vi "Calibration_user_input.vi"(4 "data mode":enum16{"Take new data point", "Refit Curve"}(ring), 6 "Mode":T4, 7 "Fixed n":bool, 8 "OK":T13, 9 "Sampling speeds":T5={"Samples /ch"=300, "Sampling Rate /ch (Hz)"=50.0} {"Sampling Rate /ch (Hz)" min=0 format="%.2f"; "Samples /ch" min=0 step=1}) -> (1 "Sampling speeds Output":T5={"Samples /ch"=300, "Sampling Rate /ch (Hz)"=50.0} {"Sampling Rate /ch (Hz)" min=0 format="%.2f"; "Samples /ch" min=0 step=1}, 2 "Fixed n out":bool, 3 "Temp (deg C)":dbl=21.0 format="%.1f", 5 "Abs Press (mbar)":dbl=1013.0 format="%.1f")   [LabVIEW 2012]
uses:
  Controls/ok_button.ctl
  Controls/Cal_Inst_type.ctl
  Calib_setup.ctl
  Controls/Ref_Inst_type.ctl
  Calib_mode.ctl
  Controls/PWA_Data.ctl
  File/Setup_Filetype.ctl
  Controls/Inst_type.ctl
  ADAM Client/Sub VIs/ADAM Controls/Channel_names.ctl
  Controls/LDA_Setup.ctl
  Controls/Setup.ctl
  Globals/Calib_global.vi
  Globals/Meas_global.vi
  Globals/LDA_meas_global_1.vi
  Globals/LDA_meas_global_2.vi
panel:
  in  "Acquisition Plug in":u16(ring) items=["ADAM_Server_Channels.vi", "DataTranslation.vi", "LDA_IP_DataTranslation.vi", "LDA_IP_NI-DAQmx.vi", "NI-DAQmx.vi", "Simulate_kernal.vi"]
  in  "PWA Data":T1
  in  "Preston tube diammeter in mm":dbl min=0.0
  in  "Reference instrument Orig":T3={"high limit (10V)"=4.0, "low limit (-10V)"=0.0, "Ch No"=4, "Off ch no"=0, "Calib filename"=path "", "Ref Instrument type"=enum."Enter Value"} {"Off ch no" min=0 max=1; "Ch No" min=0 max=7; "low limit (-10V)" min=-10 max=10 format="%.1f"; "high limit (10V)" min=-10 max=10 format="%.1f"}
  out "Message":string
  in  "Ref Instrument type":T2
  out "Info":string
  out "XW Angle Calib Present?":bool
  out "XW Velocity Calib Present?":bool
  in  "Edit temp and Press":bool
  out "2nd ref instrument":T6={"2nd Ref type"=enum."LDA", "2nd inst present"=TRUE}
  in  "Ref vel for angle calib":T7={"high limit (10V)"=6.0, "low limit (-10V)"=0.0, "Ch No"=4, "Off ch no"=0, "Calib filename"=path "", "Ref Instrument type"=enum."LDA"} {"Off ch no" min=0 max=1; "Ch No" min=0 max=50; "low limit (-10V)" min=-10 max=10 format="%.1f"; "high limit (10V)" min=-10 max=10 format="%.1f"}
  out "Instrument type":T8=enum."Cross wire angle"
  in  "angle calib":T9(ring)
  in  "Reference instrument":T7={"high limit (10V)"=4.0, "low limit (-10V)"=0.0, "Ch No"=4, "Off ch no"=0, "Calib filename"=path "", "Ref Instrument type"=enum."Enter Value"} {"Off ch no" min=0 max=1; "Ch No" min=0 max=50; "low limit (-10V)" min=-10 max=10 format="%.1f"; "high limit (10V)" min=-10 max=10 format="%.1f"}
  in  "instrument to calibrate":T10(array[cluster])=[{"high limit (10V)"=5.0, "low limit (-10V)"=3.0, "Ch No"=1, "Off ch no"=1}, {"high limit (10V)"=5.0, "low limit (-10V)"=3.0, "Ch No"=2, "Off ch no"=1}] {"Off ch no" min=0 max=1; "Ch No" min=0 max=1000; "low limit (-10V)" min=-10 max=10 format="%.3f"; "high limit (10V)" min=-10 max=10 format="%.3f"}
  in  "Instrument type":T8=enum."Pressure Transducer"
  out "Calib filename":path
  in  "Type":T11={"high limit (10V)"=4.0, "low limit (-10V)"=0.0, "Ch No"=4, "Var name"="LDA"} {"Ch No" min=0 max=7; "low limit (-10V)" min=-10 max=10 format="%.3f"; "high limit (10V)" min=-10 max=10 format="%.3f"}
  out "Ch & spans":T12(array[cluster])=[{"high limit (10V)"=5.0, "low limit (-10V)"=3.0, "Ch No"=1, "Var name"="Cross wire 1"}, {"high limit (10V)"=5.0, "low limit (-10V)"=3.0, "Ch No"=2, "Var name"="Cross wire 2"}] {"Ch No" min=0 max=7; "low limit (-10V)" min=-10 max=10 format="%.3f"; "high limit (10V)" min=-10 max=10 format="%.3f"}
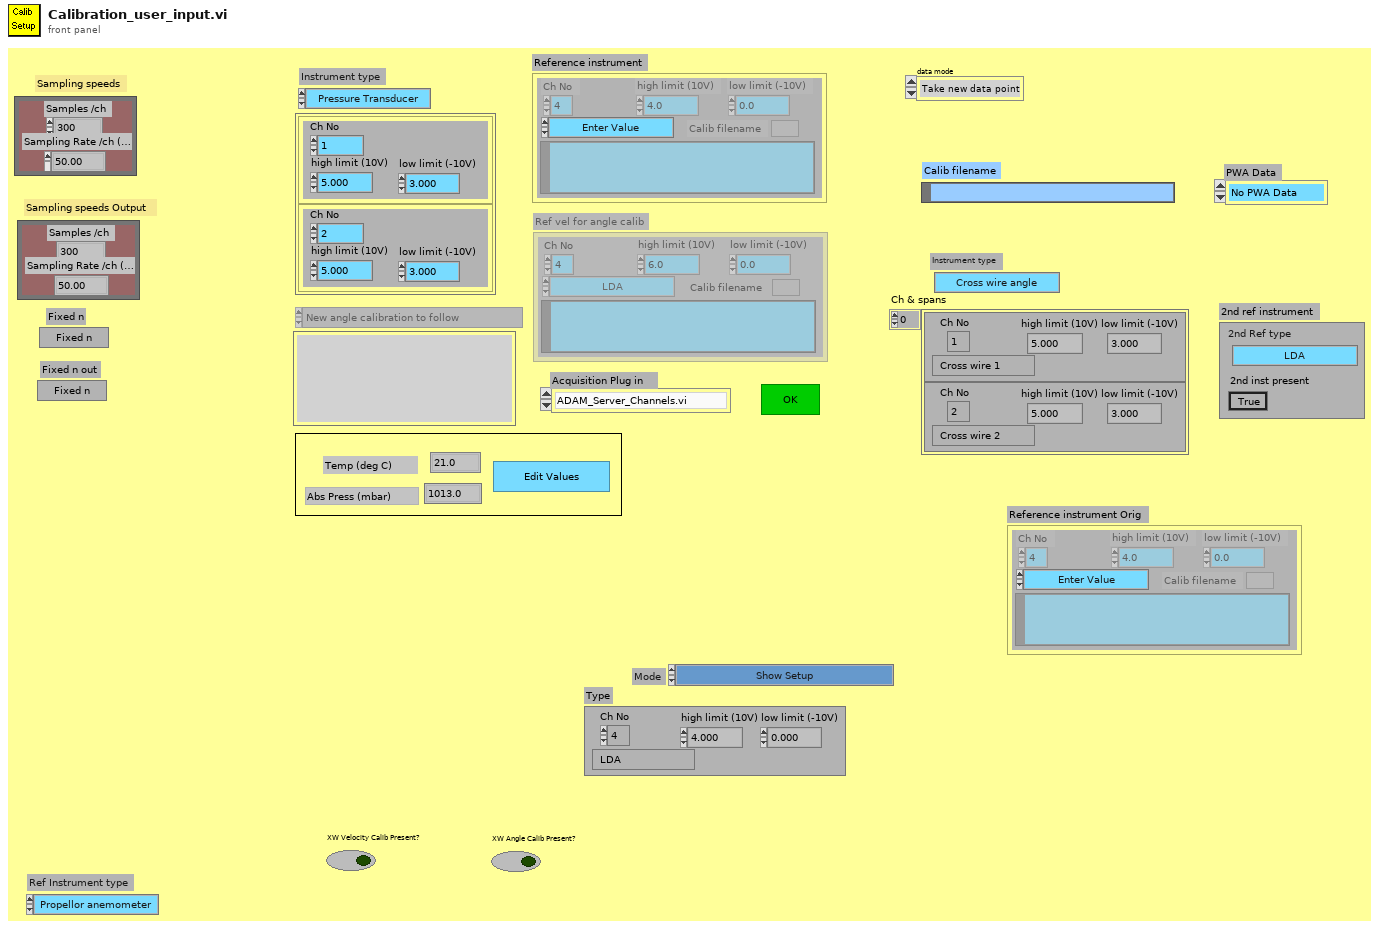
[diagram p1: front panel]
types:
  T1 = typedef "PWA_Data.ctl" = enum16{"No PWA Data", "One Ch PWA"}
  T2 = typedef "Ref_Inst_type.ctl" = enum16{"Propellor anemometer", "Pressure Transducer", "Raw voltage", "Pitot-static tube", "Preston tube", "Generic Linear", "Generic Polynomial", "Thermocouple", "LDA", "Enter Value", "ADAM Channel"}
  T3 = cluster{"high limit (10V)":sgl, "low limit (-10V)":sgl, "Ch No":i16, "Off ch no":i8, "Calib filename":path, "Ref Instrument type":T2}
  T4 = typedef "Calib_mode.ctl" = enum16{"Show Setup", "Take a New Calibration Point", "Refit Curve", "Setup Front Panel"}
  T5 = cluster{"Samples /ch":i32, "Sampling Rate /ch (Hz)":sgl}
  T6 = cluster{"2nd Ref type":T2, "2nd inst present":bool}
  T7 = typedef "Calib_setup.ctl" = cluster{"high limit (10V)":sgl, "low limit (-10V)":sgl, "Ch No":i16, "Off ch no":i8, "Calib filename":path, "Ref Instrument type":T2}
  T8 = typedef "Cal_Inst_type.ctl" = enum16{"Propeller anemometer", "Pressure Transducer", "Hot wire", "Cross wire velocity", "Cross wire angle", "Generic Linear", "Generic Polynomial", "Generic BackPoly", "Fast FID", "Thermocouple", "Cold wire", "Pulsed Wire"}
  T9 = enum16{"New angle calibration to follow", "Use the most recent angle calibration"}
  T10 = cluster{"high limit (10V)":sgl, "low limit (-10V)":sgl, "Ch No":i16, "Off ch no":i8}[]
  T11 = cluster{"high limit (10V)":sgl, "low limit (-10V)":sgl, "Ch No":i16, "Var name":string}
  T12 = cluster{"high limit (10V)":sgl, "low limit (-10V)":sgl, "Ch No":i16, "Var name":string}[]
  T13 = typedef "ok_button.ctl" = bool
  T14 = typedef "Setup_Filetype.ctl" = enum16{"Measurement Setups", "Calibration Setups", "General", "Results File Plotter Setups", "Speed Calib Tweaks"}
  T15 = typedef "Inst_type.ctl" = enum16{"Propeller anemometer", "Raw voltage", "Pressure Transducer", "Pitot-static tube", "Preston tube", "Hot wire", "Cross wire 1", "Cross wire 2", "Generic Linear", "Generic Polynomial", "Generic BackPoly", "Fast FID", "Thermocouple", "Cold wire", "Pulsed Wire", "LDA Vel", "LDA Tran time", "LDA Arr time"}
  T16 = typedef "Channel_names.ctl" = enum16{"Active Only", "Active + Off", "All Channels"}
  T17 = typedef "LDA_Setup.ctl" = cluster{"dimensions":enum16{"1D", "2D"}, "Analogue Freq Multiplier":dbl}
  T18 = typedef "Setup.ctl" = enum16{"Run Program", "Show Setup", "Save Current Setup", "Setup Front Panel"}
  T19 = cluster{"high limit (10V)":sgl, "low limit (-10V)":sgl, "Ch No":i16, "Off ch no":i8}
  T20 = typedef "BSA_Type.ctl" = enum16{"57N11", "BSA F60"}
  T21 = typedef "BSA_info_Cluster.ctl" = cluster{"GPIB Address":string, "No of Check Bytes":i32, "Extra Info":string, "COLOUR":u32, "Wavelength (nm)":dbl}
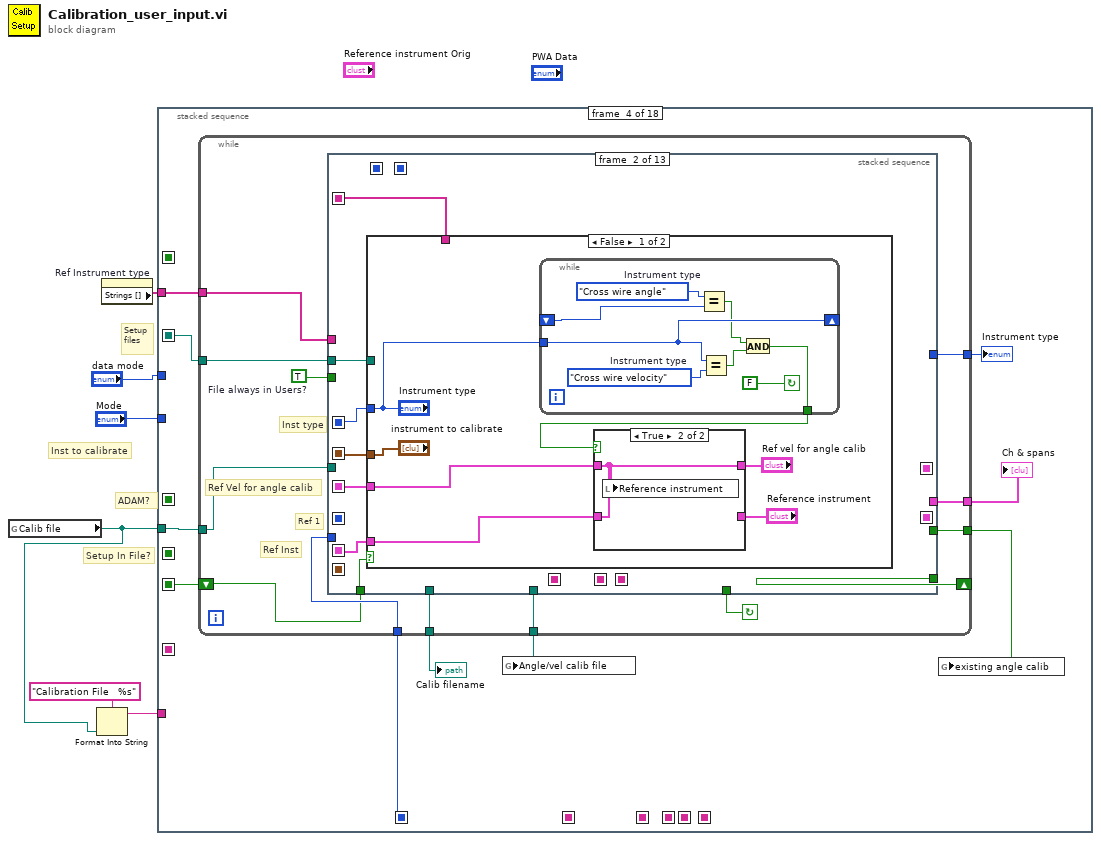
[diagram p0: block diagram]
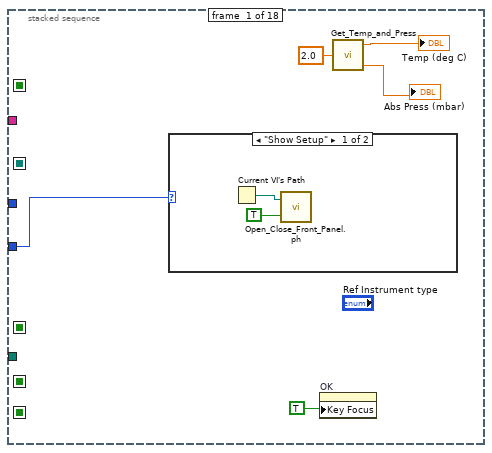
[diagram p2: hidden frame]
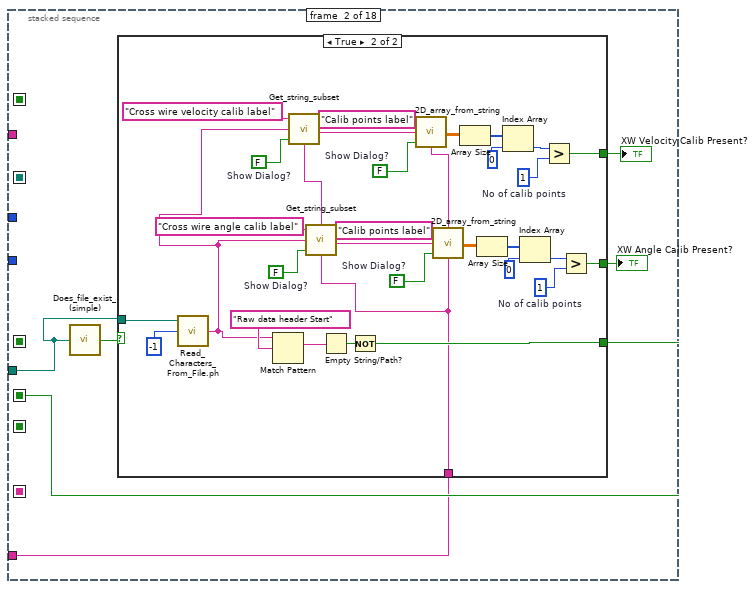
[diagram p4: hidden frame]
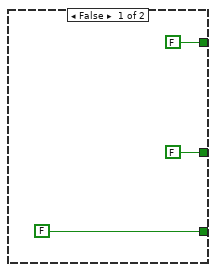
[diagram p5: hidden frame]
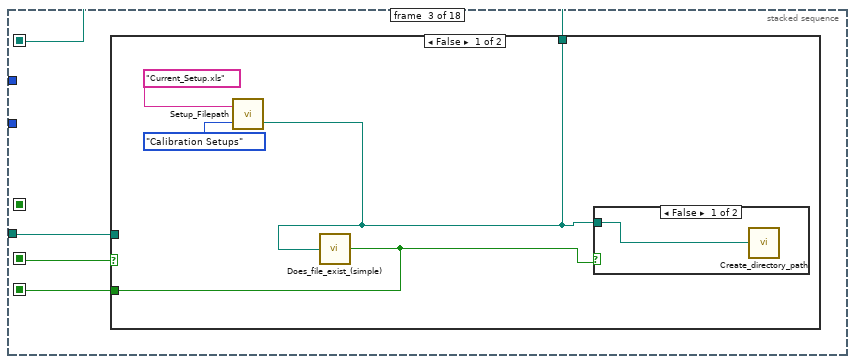
[diagram p6: hidden frame]
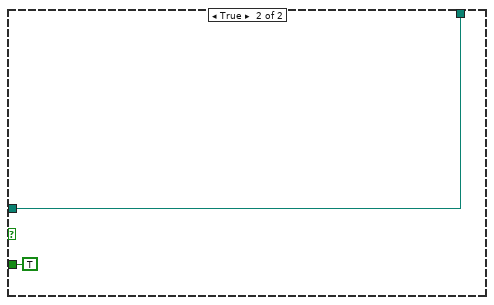
[diagram p8: hidden frame]
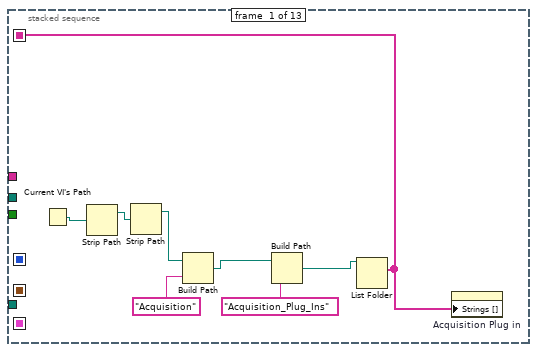
[diagram p9: hidden frame]
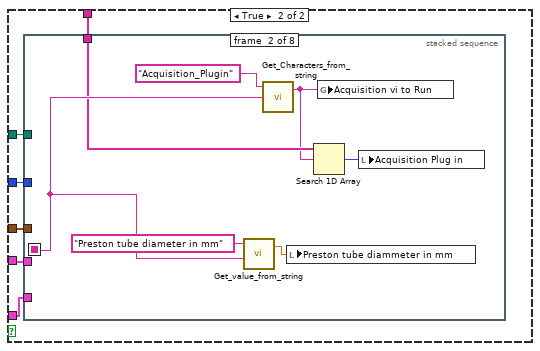
[diagram p11: hidden frame]
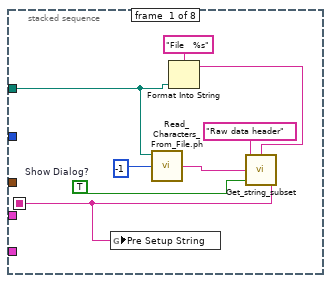
[diagram p12: hidden frame]
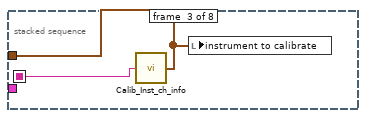
[diagram p13: hidden frame]
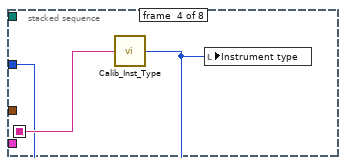
[diagram p14: hidden frame]
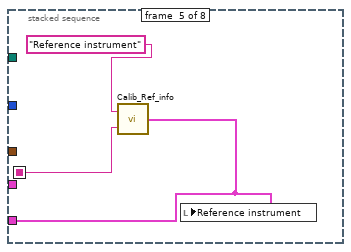
[diagram p15: hidden frame]
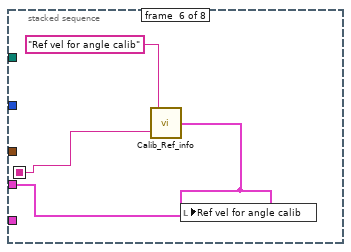
[diagram p16: hidden frame]
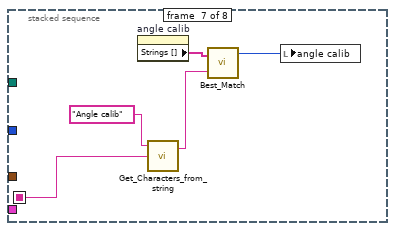
[diagram p17: hidden frame]
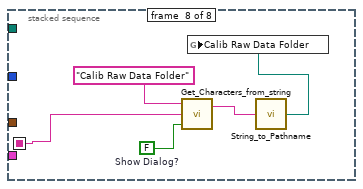
[diagram p18: hidden frame]
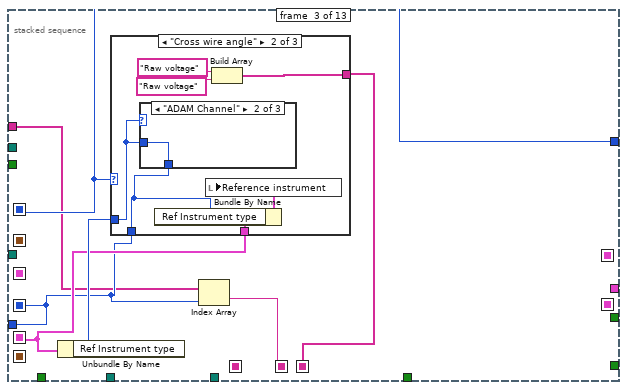
[diagram p19: hidden frame]
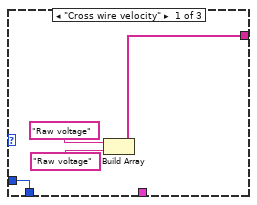
[diagram p20: hidden frame]
diagram:
  # "Inst to calibrate"
  # "Setup In File?"
  # "Setup\nfiles"
  # "ADAM?"
  n1 = global read "Calib_global.vi" "Calib file"() -> (w2:path)
  n2 = Format Into String(format string="Calibration File   %s", w2) -> (resulting string=w1:string)  [unwired: 2 in, 1 out]
  n3 = property on="Ref Instrument type" class="Enum (strict)"() -> ("Strings []"=w4:string[])  [unwired: 2 in, 2 out]
  n4 = stacked-sequence {
    seq-local: [_ _ w55 _ _ _ _ _ _ _ _ _ _ _ _ _ _ _] -> [_ _ _ w71 _ _ _ _ _ _ _ _ _ _ _ _ _ _]
    seq-local: [_ _ w56 _ _ _ _ _ _ _ _ _ _ _ _ _ _ _] -> [_ _ _ w69 _ _ _ _ _ _ _ _ _ _ _ _ _ _]
    seq-local: [_ _ _ w68 _ _ _ _ _ _ _ _ _ _ _ _ _ _] -> [_ _ _ _ _ _ _ w612 _ _ _ _ _ _ _ _ _ _]
    seq-local: [_ _ _ _ _ _ _ w613 _ _ _ _ _ _ _ _ _ _] -> [_ _ _ _ _ _ _ _ w630 _ _ _ _ _ _ _ _ _]
    seq-local: [_ _ _ _ _ _ _ _ w633 _ _ _ _ _ _ _ _ _] -> [_ _ _ _ _ _ _ _ _ _ _ _ _ _ w809 _ _ _]
    seq-local: [_ _ _ _ _ _ _ _ _ _ w722 _ _ _ _ _ _ _] -> [_ _ _ _ _ _ _ _ _ _ _ _ _ _ w808 _ w846 _]
    seq-local: [_ _ _ _ _ _ _ _ _ _ w719 _ _ _ _ _ _ _] -> [_ _ _ _ _ _ _ _ _ _ _ _ _ _ _ w815 _ _]
    seq-local: [_ w19 _ _ _ _ _ _ _ _ _ _ _ _ _ _ _ _] -> [_ _ w54 _ _ _ _ _ _ _ _ _ _ _ _ _ _ _]
    seq-local: [_ _ _ _ _ _ _ _ _ _ _ w734 _ _ _ _ _ _] -> [_ _ _ _ _ _ _ _ _ _ _ _ _ _ w801 _ _ _]
    seq-local: [_ _ _ _ _ _ _ _ _ _ _ _ _ w759 _ _ _ _] -> [_ _ _ _ _ _ _ _ _ _ _ _ _ _ w789 _ _ _]
    seq-local: [_ _ _ _ _ _ _ _ _ _ _ _ w741 _ _ _ _ _] -> [_ _ _ _ _ _ _ _ _ _ _ _ _ _ w785 _ w836 _]
    seq-local: [_ _ _ _ _ _ _ _ _ w668 _ _ _ _ _ _ _ _] -> [_ _ _ _ _ _ _ _ _ _ _ _ _ _ w784 _ _ _]
    tunnel: "Mode" -> [w7 _ _ _ w535 w553 _ _ w632 w681 _ _ w742 _ _ w817 _ w863]
    tunnel: "data mode" -> [_ _ _ _ w529 _ _ _ _ _ _ _ _ _ _ _ _ _]
    tunnel: w2 -> [_ w17 w53 w65 _ _ _ _ _ _ _ _ _ _ _ _ _ _]
    tunnel: w4 -> [_ _ _ w64 _ _ _ _ _ _ _ _ _ _ _ _ _ _]
    tunnel: w1 -> [_ w14 _ _ _ _ _ _ _ _ _ _ _ _ _ _ _ _]
    frame #0 {
      n5 = case shown="\"Show Setup\"" w7 {
        frame "Show Setup" {
          n6 = Current VI's Path() -> (path=w13:path)
          n7 = call "Open_Close_Front_Panel.ph.vi"("Front Panel Window:Open"=TRUE, "VI path"=w13) -> ()  [unwired: 2 out]
        }
        frame "Take a New Calibration Point", Default {
        }
      }
      n8 = property on="OK" class="Bool"("Key Focus"=TRUE) -> ()  [unwired: 2 in, 2 out]
      n9 = call "Get_Temp_and_Press.vi"("Averaging time (mins)"=2.0) -> ("Abs Press (mbar)"=→"Abs Press (mbar)":dbl, "Temperature"=→"Temp (deg C)":dbl)  [unwired: 3 out]
    }
    frame #1 {
      n10 = call "Does_file_exist_(simple).vi"("Pathname"=w17) -> ("exists?"=w18:bool)
      n11 = case shown="True" w18 {
        tunnel: [FALSE w48] -> w19
        tunnel: w17 -> [_ w47]
        tunnel: [FALSE w25] -> w16
        tunnel: [FALSE w24] -> w15
        tunnel: w14 -> [_ w23]
        frame False {
        }
        frame True {
          w36 = 1  # No of calib points
          w30 = FALSE  # Show Dialog?
          w28 = FALSE  # Show Dialog?
          w37 = 1  # No of calib points
          w43 = FALSE  # Show Dialog?
          w45 = FALSE  # Show Dialog?
          n12 = call "Read_Characters_From_File.ph.vi"("file path (dialog if empty)"=w47, "number of characters (all:-1)"=-1) -> ("character string"=w26:string)  [unwired: 7 out]
          n13 = Match Pattern(string=w26, regular expression="Raw data header Start") -> (match substring=w50:string)  [unwired: 4 out]
          n14 = call "Get_string_subset.vi"("String Name"=w23, "Show Dialog?"=w28, "String to split"=w26, "File Label"="Cross wire velocity calib label") -> ("Output string"=w34:string)  [unwired: 1 out]
          n15 = call "Get_string_subset.vi"("String Name"=w23, "Show Dialog?"=w45, "String to split"=w26, "File Label"="Cross wire angle calib label") -> ("Output string"=w39:string)  [unwired: 1 out]
          n16 = Empty String/Path?(string/path=w50) -> (empty?=w49:bool)
          n17 = Not(x=w49) -> (.not. x?=w48:bool)
          n18 = call "2D_array_from_string.vi"("String Name"=w23, "Show Dialog?"=w30, "Input string"=w34, "Array title"="Calib points label") -> ("2D data array"=w31:dbl[][])
          n19 = call "2D_array_from_string.vi"("String Name"=w23, "Show Dialog?"=w43, "Input string"=w39, "Array title"="Calib points label") -> ("2D data array"=w42:dbl[][])
          n20 = Array Size(array=w31) -> (size(s)=w32:i32[])
          n21 = Array Size(array=w42) -> (size(s)=w41:i32[])
          n22 = Index Array(array=w32, index=0 ("Index")) -> (element=w35:i32)
          n23 = Index Array(array=w41, index=0 ("Index")) -> (element=w38:i32)
          n24 = Greater?(x=w35, y=w36) -> (0:w24:bool)
          n25 = Greater?(x=w38, y=w37) -> (0:w25:bool)
        }
      }
      "XW Velocity Calib Present?" <- w15
      "XW Angle Calib Present?" <- w16
    }
    frame #2 {
      n26 = case shown="False" w54 {
        tunnel: [w60 TRUE ("exists")] -> w56
        tunnel: [w57 w63] -> w55
        tunnel: w53 -> [_ w63]
        frame False {
          n27 = call "Setup_Filepath.vi"("Setup File Type"=Setup_Filetype."Calibration Setups", "Filename in"="Current_Setup.xls") -> ("Filename Out"=w57:path)  [unwired: 1 out]
          n28 = call "Does_file_exist_(simple).vi"("Pathname"=w57) -> ("exists?"=w60:bool)
          n29 = case shown="False" w60 {
            tunnel: w57 -> [w61 _]
            frame False {
              n30 = call "Create_directory_path.vi"("Path name"=w61) -> ()  [unwired: 1 in, 2 out]
            }
            frame True {
            }
          }
        }
        frame True {
        }
      }
    }
    frame #3 {
      n31 = while {
        tunnel: w64 -> [w77]
        shift-left: w69 -> [w80]
        shift-right: [w79] -> _
        tunnel: [w81] -> w70
        tunnel: w71 -> [w82]
        tunnel: [w83] -> w67
        tunnel: [w84] -> w73
        tunnel: [w85] -> w68
        tunnel: [w86] -> w72
        tunnel: [w75] -> w66
        tunnel: w65 -> [w74]
        stop <- w78 continue-if-true
        w76 = TRUE  # File always in Users?
        # "Ref 1"
        # "Ref Inst"
        # "Ref Vel for angle calib"
        # "Inst type"
        n32 = stacked-sequence {
          seq-local: [_ _ w163 _ _ _ _ _ _ _ _ _ _] -> [_ _ _ _ _ w279 _ _ _ _ _ _ _]
          seq-local: [_ _ w167 _ _ _ _ _ _ _ _ _ _] -> [_ _ _ _ _ _ _ _ w430 _ _ _ _]
          seq-local: [_ _ _ _ _ w273 _ _ _ _ _ _ _] -> [_ _ _ _ _ _ _ _ _ w447 _ _ _]
          seq-local: [_ _ w162 _ _ _ _ _ _ _ _ _ _] -> [_ _ _ _ _ _ _ _ _ w445 _ _ _]
          seq-local: [_ _ _ _ _ _ _ _ w429 _ _ _ _] -> [_ _ _ _ _ _ _ _ _ w446 _ _ _]
          seq-local: [_ _ _ _ _ _ _ w351 _ _ _ _ _] -> [_ _ _ _ _ _ _ _ _ w442 _ _ _]
          seq-local: [_ _ _ _ _ _ w347 _ _ _ _ _ _] -> [_ _ _ _ _ _ _ _ _ w441 _ _ _]
          seq-local: [_ w99 _ _ _ _ _ _ _ _ _ _ _] -> [_ _ w165 w190 w203 _ _ w352 _ _ _ _ _]
          seq-local: [_ w98 _ _ _ _ _ _ _ _ _ _ _] -> [_ _ _ w189 _ _ _ _ _ _ _ _ _]
          seq-local: [_ w97 _ _ _ _ _ _ _ _ _ _ _] -> [_ _ _ _ _ _ w349 w353 _ w440 _ _ _]
          seq-local: [_ w96 _ _ _ _ _ _ _ _ _ _ _] -> [_ _ w164 _ _ _ _ _ _ w439 _ _ w525]
          seq-local: [_ _ _ _ _ _ _ _ _ w438 _ _ _] -> [_ _ _ _ _ _ _ _ _ _ _ w484 _]
          seq-local: [_ _ _ w185 _ _ _ _ _ _ _ _ _] -> [_ _ _ _ _ _ _ _ w428 _ _ _ _]
          seq-local: [w87 _ _ _ _ _ _ _ _ _ _ _ _] -> [_ w95 _ _ _ _ _ _ _ _ _ _ _]
          tunnel: [_ _ _ _ _ _ _ _ _ w444 _ _ _] -> w86
          tunnel: [_ _ w163 _ _ _ _ _ _ _ _ _ _] -> w85
          tunnel: [_ _ _ _ _ _ _ _ _ w438 _ _ _] -> w84
          tunnel: [_ _ _ _ w208 _ _ _ _ _ _ _ _] -> w83
          tunnel: w82 -> [_ w101 _ _ _ _ _ _ _ _ _ _ _]
          tunnel: [_ _ w165 _ _ _ _ _ _ _ _ _ _] -> w81
          tunnel: w80 -> [_ w100 _ _ _ _ _ _ _ _ _ _ _]
          tunnel: [_ _ _ _ _ _ _ _ _ _ _ FALSE _] -> w79
          tunnel: [_ _ _ _ _ _ _ _ _ _ _ w482 _] -> w78
          tunnel: w77 -> [_ _ w161 _ _ _ w346 _ _ _ _ _ _]
          tunnel: w76 -> [_ _ _ _ _ _ _ _ _ _ _ _ _]
          tunnel: [_ _ _ _ w207 _ _ _ _ _ _ _ _] -> w75
          tunnel: w74 -> [_ _ _ _ w209 _ _ _ _ _ _ _ _]
          frame #0 {
            n33 = Current VI's Path() -> (path=w90:path)
            n34 = Strip Path(path=w90) -> (stripped path=w89:path)  [unwired: 1 out]
            n35 = Strip Path(path=w89) -> (stripped path=w88:path)  [unwired: 1 out]
            n36 = Build Path(base path=w88, name or relative path="Acquisition") -> (appended path=w93:path)
            n37 = Build Path(base path=w93, name or relative path="Acquisition_Plug_Ins") -> (appended path=w94:path)
            n38 = List Folder(path=w94) -> (filenames=w87:string[])  [unwired: 3 in, 3 out]
            n39 = property on="Acquisition Plug in" class="Ring (strict)"("Strings []"=w87) -> ()  [unwired: 2 in, 2 out]
          }
          frame #1 {
            n40 = case shown="False" w100 {
              tunnel: w101 -> [_ w125]
              tunnel: ["Instrument type" w123] -> w99
              tunnel: ["instrument to calibrate" w124] -> w98
              tunnel: [w103 w121] -> w97
              tunnel: [w105 w122] -> w96
              tunnel: w95 -> [_ w120]
              frame False {
                n41 = while {
                  shift-right: [w117] -> _
                  shift-left: _ -> [w115]
                  tunnel: "Instrument type" -> [w117]
                  tunnel: [w112] -> w106
                  stop <- FALSE continue-if-true
                  w116 = Cal_Inst_type."Cross wire angle"  # Instrument type
                  w118 = Cal_Inst_type."Cross wire velocity"  # Instrument type
                  n42 = Equal?(x=w116, y=w115) -> (x = y?=w113:bool)
                  n43 = Equal?(x=w117, y=w118) -> (x = y?=w114:bool)
                  n44 = And(x=w113, y=w114) -> (x .and. y?=w112:bool)
                }
                n45 = case shown="True" w106 {
                  tunnel: [w110 w111] -> w105
                  tunnel: "Reference instrument" -> [w110 _]
                  tunnel: [w109 w111] -> w103
                  tunnel: "Ref vel for angle calib" -> [w109 w111]
                  frame False {
                  }
                  frame True {
                    n46 = local write "Reference instrument"(w111) -> ()
                  }
                }
              }
              frame True {
                n47 = stacked-sequence {
                  seq-local: [w130 _ _ _ _ _ _ _] -> [_ w137 w142 w144 w146 w149 w153 w158]
                  tunnel: w125 -> [w127 _ _ _ _ _ _ _]
                  tunnel: [_ _ w141 _ _ _ _ _] -> w124
                  tunnel: [_ _ _ w143 _ _ _ _] -> w123
                  tunnel: [_ _ _ _ w145 _ _ _] -> w122
                  tunnel: [_ _ _ _ _ w148 _ _] -> w121
                  tunnel: w120 -> [_ w136 _ _ _ _ _ _]
                  frame #0 {
                    w129 = TRUE  # Show Dialog?
                    n48 = call "Read_Characters_From_File.ph.vi"("file path (dialog if empty)"=w127, "number of characters (all:-1)"=-1) -> ("character string"=w133:string)  [unwired: 7 out]
                    n49 = Format Into String(format string="File   %s", w127) -> (resulting string=w126:string)  [unwired: 2 in, 1 out]
                    n50 = call "Get_string_subset.vi"("String Name"=w126, "Show Dialog?"=w129, "String to split"=w133, "File Label"="Raw data header") -> ("Output string"=w130:string)  [unwired: 1 out]
                    n51 = global write "Calib_global.vi" "Pre Setup String"(w130) -> ()
                  }
                  frame #1 {
                    n52 = call "Get_value_from_string.vi"("Input string"=w137, "Variable name"="Preston tube diameter in mm") -> ("Value"=w139:dbl)  [unwired: 1 in, 1 out]
                    n53 = call "Get_Characters_from_string.vi"("Input string"=w137, "Variable name"="Acquisition_Plugin") -> ("Value"=w135:string)  [unwired: 1 in, 1 out]
                    n54 = local write "Preston tube diammeter in mm"(w139) -> ()
                    n55 = Search 1D Array(1D array=w136, element=w135) -> (index of element=w134:i32)  [unwired: 1 out]
                    n56 = global write "Meas_global.vi" "Acquisition vi to Run"(w135) -> ()
                    n57 = local write "Acquisition Plug in"(w134) -> ()
                  }
                  frame #2 {
                    n58 = call "Calib_Inst_ch_info.vi"("Input string"=w142) -> ("instrument to calibrate"=w141:T10)
                    n59 = local write "instrument to calibrate"(w141) -> ()
                  }
                  frame #3 {
                    n60 = call "Calib_Inst_Type.vi"("Input string"=w144) -> ("Instrument type"=w143:T8)
                    n61 = local write "Instrument type"(w143) -> ()
                  }
                  frame #4 {
                    n62 = call "Calib_Ref_info.vi"("Input string"=w146, "Reference Name"="Reference instrument") -> ("Reference instrument"=w145:T7)
                    n63 = local write "Reference instrument"(w145) -> ()
                  }
                  frame #5 {
                    n64 = call "Calib_Ref_info.vi"("Input string"=w149, "Reference Name"="Ref vel for angle calib") -> ("Reference instrument"=w148:T7)
                    n65 = local write "Ref vel for angle calib"(w148) -> ()
                  }
                  frame #6 {
                    n66 = property on="angle calib" class="Enum (strict)"() -> ("Strings []"=w155:string[])  [unwired: 2 in, 2 out]
                    n67 = call "Get_Characters_from_string.vi"("Input string"=w153, "Variable name"="Angle calib") -> ("Value"=w152:string)  [unwired: 1 in, 1 out]
                    n68 = call "Best_Match.vi"("Input String"=w152, "String Options"=w155) -> ("index of element"=w151:i32)  [unwired: 1 out]
                    n69 = local write "angle calib"(w151) -> ()
                  }
                  frame #7 {
                    w159 = FALSE  # Show Dialog?
                    n70 = call "Get_Characters_from_string.vi"("Show Dialog?"=w159, "Input string"=w158, "Variable name"="Calib Raw Data Folder") -> ("Value"=w157:string)  [unwired: 1 out]
                    n71 = call "String_to_Pathname.vi"("Input String"=w157) -> ("path"=w156:path)
                    n72 = global write "Calib_global.vi" "Calib Raw Data Folder"(w156) -> ()
                  }
                }
              }
            }
          }
          frame #2 {
            n73 = Unbundle By Name(w164) -> ("Ref Instrument type"=w166:T2)
            n74 = case shown="\"Cross wire angle\"" w165 {
              tunnel: [w170 w178 w183] -> w167
              tunnel: w166 -> [w168 w172 w182]
              tunnel: [w168 w175 w182] -> w163
              tunnel: w164 -> [_ w176 _]
              frame "Cross wire velocity" {
                n75 = Build Array("Raw voltage", "Raw voltage") -> (w170:string[])
              }
              frame "Cross wire angle" {
                n76 = case shown="\"ADAM Channel\"" w172 {
                  tunnel: [w179 w180 Ref_Inst_type."Enter Value" ("Ref Instrument type")] -> w175
                  tunnel: w172 -> [w179 w180 _]
                  frame "Enter Value" {
                  }
                  frame "ADAM Channel" {
                  }
                  frame "LDA", Default {
                  }
                }
                n77 = Bundle By Name(cluster=w176, "Ref Instrument type"=w175) -> (w177:T7)
                n78 = local write "Reference instrument"(w177) -> ()
                n79 = Build Array("Raw voltage", "Raw voltage") -> (w178:string[])
              }
              frame "Generic Linear", Default {
                n80 = Build Array("Raw voltage") -> (w183:string[])
              }
            }
            n81 = Index Array(array=w161, index=w163) -> (element=w162:string)
          }
          frame #3 {
            n82 = Array Size(array=w189) -> (size(s)=w188:i32)
            n83 = case shown="\"Pulsed Wire\"" w190 {
              tunnel: [2 2 1 0] -> w187
              frame "Cross wire velocity" {
              }
              frame "Cross wire angle" {
              }
              frame "Generic Linear", Default {
              }
              frame "Pulsed Wire" {
              }
            }
            n84 = Equal?(x=w187, y=w188) -> (x = y?=w186:bool)
            n85 = case shown="False" w186 {
              tunnel: w187 -> [w196 _]
              tunnel: w189 -> [w192 w198]
              tunnel: [w191 w198] -> w185
              frame False {
                n86 = Index Array(array=w192, index=0) -> (element=w193:T19)
                n87 = Build Array (concatenate)(w192, w193) -> (w195:T10)
                n88 = for {
                  N: w196 -> [_]
                  tunnel: w195 -> [w197] mode=indexing
                  tunnel: [w197] -> w191 mode=indexing
                }
                n89 = local write "instrument to calibrate"(w191) -> ()
              }
              frame True {
              }
            }
          }
          frame #4 {
            n90 = case shown="\"Cross wire velocity\"" w203 {
              tunnel: w209 -> [_ w220 w242]
              tunnel: [path "" w221 w243] -> w208
              tunnel: [FALSE w219 w241] -> w207
              tunnel: [w210 w215 w237] -> w206
              tunnel: [w212 w218 w240] -> w205
              tunnel: ["" w217 w238] -> w204
              tunnel: w203 -> [_ w216 w239]
              frame "Propeller anemometer", Default {
                w210 = u8 2  # Disabled
                w212 = u8 2  # Disabled
              }
              frame "Cross wire angle" {
                w215 = u8 0  # Disabled
                w218 = u8 2  # Disabled
                n91 = local read "XW Velocity Calib Present?"() -> (w222:bool)
                n92 = case shown="False" w222 {
                  tunnel: [w226 w236] -> w221
                  tunnel: w220 -> [_ w236]
                  tunnel: [TRUE TRUE] -> w219
                  tunnel: [w224 w234] -> w217
                  tunnel: w216 -> [w223 _]
                  frame False {
                    w230 = 0  # index
                    n93 = local read "instrument to calibrate"() -> (w231:T10)
                    n94 = Index Array(array=w231, index=w230) -> (element=w229:T19)
                    n95 = Unbundle By Name(w229) -> ("Ch No"=w227:i16)
                    n96 = call "XW_file_info.vi"("Instrument type"=w223, "Ch No"=w227) -> ("Filename"=w226:path, "resulting string"=w224:string, "File Exists?"=w225:bool)
                    n97 = case shown="False" w225 {
                      frame False {
                        w232 = Cal_Inst_type."Cross wire velocity"  # Instrument type
                        w233 = "You need to do a velocity calibration before you can do the angle calibration"  # message
                        n98 = local write "Instrument type"(w232) -> ()
                        n99 = One Button Dialog(message=w233) -> ()  [unwired: 2 out]
                      }
                      frame True {
                      }
                    }
                  }
                  frame True {
                    w234 = "Will use the velocity Calibration info already in the Calibration file. "  # resulting string
                  }
                }
              }
              frame "Cross wire velocity" {
                w237 = u8 2  # Disabled
                n100 = local read "XW Angle Calib Present?"() -> (w244:bool)
                n101 = case shown="False" w244 {
                  tunnel: [w253 w272] -> w243
                  tunnel: w242 -> [_ w272]
                  tunnel: [TRUE FALSE] -> _
                  tunnel: [w252 TRUE] -> w241
                  tunnel: [w251 w269] -> w240
                  tunnel: w239 -> [w249 _]
                  tunnel: [w246 w268] -> w238
                  frame False {
                    w257 = 0  # index
                    n102 = local read "instrument to calibrate"() -> (w258:T10)
                    n103 = Index Array(array=w258, index=w257) -> (element=w256:T19)
                    n104 = Unbundle By Name(w256) -> ("Ch No"=w250:i16)
                    n105 = call "XW_file_info.vi"("Instrument type"=w249, "Ch No"=w250) -> ("Filename"=w248:path, "resulting string"=w245:string, "File Exists?"=w247:bool)
                    n106 = case shown="\"New angle calibration to follow\"" "angle calib" {
                      tunnel: [path "" w264] -> w253
                      tunnel: w248 -> [_ w264]
                      tunnel: [FALSE TRUE] -> w252
                      tunnel: ["This XW velocity Calibration MUST be followed by an angle calibration, before XW measurements can be made." w262] -> w246
                      tunnel: w245 -> [_ w262]
                      frame "New angle calibration to follow" {
                      }
                      frame "Use the most recent angle calibration" {
                      }
                    }
                    n107 = case shown="False" w247 {
                      tunnel: [w265 w267] -> w251
                      frame False {
                        w265 = u8 2  # Disabled
                        w266 = T9."New angle calibration to follow"  # angle calib
                        n108 = local write "angle calib"(w266) -> ()
                      }
                      frame True {
                        w267 = u8 0  # Disabled
                      }
                    }
                  }
                  frame True {
                    w268 = "Will use the angle Calibration info already in the Calibration file. "  # resulting string
                    w269 = u8 0  # Disabled
                  }
                }
              }
            }
            "Info" <- w204
            n109 = property on="Ref vel for angle calib" class="Clust (strict)"("Disabled"=w206) -> ()  [unwired: 2 in, 2 out]
            n110 = property on="angle calib" class="Enum (strict)"("Disabled"=w205) -> ()  [unwired: 2 in, 2 out]
          }
          frame #5 {
            n111 = case shown="\"Enter Value\"" w279 {
              tunnel: [u8 0 u8 0 u8 0 u8 0 u8 0 u8 0 u8 0 u8 2 u8 2 u8 2 u8 2] -> w274
              tunnel: [u8 0 u8 0 u8 2 u8 0 u8 0 u8 0 u8 0 u8 2 u8 2 u8 2 u8 2] -> w278
              tunnel: [u8 0 u8 0 u8 0 u8 0 u8 0 u8 0 u8 0 u8 2 u8 2 u8 2 u8 2] -> w277
              tunnel: [u8 0 u8 0 u8 0 u8 0 u8 0 u8 0 u8 0 u8 2 u8 2 u8 2 u8 2] -> w276
              tunnel: [u8 0 u8 0 u8 0 u8 0 u8 0 u8 0 u8 0 u8 2 u8 2 u8 2 u8 2] -> w275
              tunnel: [1 1 1 1 1 1 1 0 0 0 0] -> w273
              frame "Propellor anemometer" {
              }
              frame "Pressure Transducer" {
              }
              frame "Raw voltage" {
              }
              frame "Pitot-static tube" {
              }
              frame "Preston tube" {
              }
              frame "Generic Linear" {
              }
              frame "Generic Polynomial" {
              }
              frame "Thermocouple" {
              }
              frame "LDA" {
              }
              frame "Enter Value" {
              }
              frame "ADAM Channel" {
              }
            }
            n112 = property on="Calib filename" class="Path"("Disabled"=w278) -> ()  [unwired: 2 in, 2 out]
            n113 = property on="Ch No" class="DigNum (strict)"("Disabled"=w277) -> ()  [unwired: 2 in, 2 out]
            n114 = property on="high limit (10V)" class="DigNum (strict)"("Disabled"=w276) -> ()  [unwired: 2 in, 2 out]
            n115 = property on="low limit (-10V)" class="DigNum (strict)"("Disabled"=w275) -> ()  [unwired: 2 in, 2 out]
            n116 = property on="Off ch no" class="DigNum (strict)"("Disabled"=w274) -> ()  [unwired: 2 in, 2 out]
          }
          frame #6 {
            n117 = Unbundle By Name(w349) -> ("Ref Instrument type"=w348:T2)
            n118 = Index Array(array=w346, index=w348) -> (element=w347:string)
          }
          frame #7 {
            n119 = Unbundle By Name(w353) -> ("Ref Instrument type"=w354:T2)
            n120 = case shown="\"ADAM Channel\"" w354 {
              tunnel: [u8 0 u8 0 u8 0 u8 0 u8 0 u8 0 u8 0 u8 0 u8 2 u8 2 u8 2] -> w355
              tunnel: [u8 0 u8 0 u8 2 u8 0 u8 0 u8 0 u8 0 u8 0 u8 2 u8 2 u8 2] -> w359
              tunnel: [u8 0 u8 0 u8 0 u8 0 u8 0 u8 0 u8 0 u8 0 u8 2 u8 2 u8 2] -> w358
              tunnel: [u8 0 u8 0 u8 0 u8 0 u8 0 u8 0 u8 0 u8 0 u8 2 u8 2 u8 2] -> w357
              tunnel: [u8 0 u8 0 u8 0 u8 0 u8 0 u8 0 u8 0 u8 0 u8 2 u8 2 u8 2] -> w356
              tunnel: [enum16{"No 2nd ref inst", "Add 2nd ref inst"}."Add 2nd ref inst" enum16{"No 2nd ref inst", "Add 2nd ref inst"}."Add 2nd ref inst" enum16{"No 2nd ref inst", "Add 2nd ref inst"}."Add 2nd ref inst" enum16{"No 2nd ref inst", "Add 2nd ref inst"}."Add 2nd ref inst" enum16{"No 2nd ref inst", "Add 2nd ref inst"}."Add 2nd ref inst" enum16{"No 2nd ref inst", "Add 2nd ref inst"}."Add 2nd ref inst" enum16{"No 2nd ref inst", "Add 2nd ref inst"}."Add 2nd ref inst" enum16{"No 2nd ref inst", "Add 2nd ref inst"}."Add 2nd ref inst" enum16{"No 2nd ref inst", "Add 2nd ref inst"}."No 2nd ref inst" enum16{"No 2nd ref inst", "Add 2nd ref inst"}."No 2nd ref inst" enum16{"No 2nd ref inst", "Add 2nd ref inst"}."No 2nd ref inst"] -> w350
              frame "Propellor anemometer" {
              }
              frame "Pressure Transducer" {
              }
              frame "Raw voltage" {
              }
              frame "Pitot-static tube" {
              }
              frame "Preston tube" {
              }
              frame "Generic Linear" {
              }
              frame "Generic Polynomial" {
              }
              frame "Thermocouple" {
              }
              frame "LDA" {
              }
              frame "Enter Value" {
              }
              frame "ADAM Channel" {
              }
            }
            n121 = case shown="\"Cross wire angle\"" w352 {
              tunnel: [w360 enum16{"No 2nd ref inst", "Add 2nd ref inst"}."No 2nd ref inst"] -> w351
              tunnel: w350 -> [w360 _]
              frame "Cross wire angle" {
              }
              frame "Generic Linear", Default {
              }
            }
            n122 = property on="Calib filename" class="Path"("Disabled"=w359) -> ()  [unwired: 2 in, 2 out]
            n123 = property on="low limit (-10V)" class="DigNum (strict)"("Disabled"=w358) -> ()  [unwired: 2 in, 2 out]
            n124 = property on="high limit (10V)" class="DigNum (strict)"("Disabled"=w357) -> ()  [unwired: 2 in, 2 out]
            n125 = property on="Ch No" class="DigNum (strict)"("Disabled"=w356) -> ()  [unwired: 2 in, 2 out]
            n126 = property on="Off ch no" class="DigNum (strict)"("Disabled"=w355) -> ()  [unwired: 2 in, 2 out]
          }
          frame #8 {
            n127 = for {
              tunnel: w430 -> [w437] mode=indexing
              tunnel: [w435] -> w429 mode=indexing
              tunnel: w428 -> [w431] mode=indexing
              n128 = Unbundle By Name(w431) -> ("high limit (10V)"=w434:sgl, "low limit (-10V)"=w433:sgl, "Ch No"=w432:i16)
              n129 = Bundle By Name(cluster="Type", "high limit (10V)"=w434, "low limit (-10V)"=w433, "Ch No"=w432, "Var name"=w437) -> (w435:T11)
            }
          }
          frame #9 {
            n130 = local read "Type"() -> (w443:T11)
            n131 = case shown="..0" w447 {
              tunnel: [w451 w473] -> w438
              tunnel: w446 -> [w454 w467]
              tunnel: w439 -> [_ w470]
              tunnel: w445 -> [_ w469]
              tunnel: [w453 w472] -> w444
              tunnel: w443 -> [w452 w471]
              tunnel: w440 -> [w448 _]
              tunnel: w442 -> [w450 _]
              tunnel: w441 -> [w449 _]
              frame ..0 {
                n132 = case shown="\"No 2nd ref inst\"" w450 {
                  tunnel: [w456 w466] -> w451
                  tunnel: w449 -> [_ w465]
                  tunnel: w448 -> [_ w464]
                  tunnel: w452 -> [_ w463]
                  tunnel: [path "" w462] -> w453
                  tunnel: w454 -> [w456 w457]
                  frame "No 2nd ref inst" {
                  }
                  frame "Add 2nd ref inst" {
                    n133 = Unbundle By Name(w464) -> ("high limit (10V)"=w459:sgl, "low limit (-10V)"=w460:sgl, "Ch No"=w461:i16, "Calib filename"=w462:path)
                    n134 = Bundle By Name(cluster=w463, "high limit (10V)"=w459, "low limit (-10V)"=w460, "Ch No"=w461, "Var name"=w465) -> (w458:T11)
                    n135 = Build Array (concatenate)(w458, w457) -> (w466:T12)
                  }
                }
              }
              frame 1.. {
                n136 = Unbundle By Name(w470) -> ("high limit (10V)"=w476:sgl, "low limit (-10V)"=w475:sgl, "Ch No"=w474:i16, "Calib filename"=w472:path)
                n137 = Bundle By Name(cluster=w471, "high limit (10V)"=w476, "low limit (-10V)"=w475, "Ch No"=w474, "Var name"=w469) -> (w468:T11)
                n138 = local write "Type"(w468) -> ()
                n139 = Build Array (concatenate)(w468, w467) -> (w473:T12)
              }
            }
          }
          frame #10 {
            n140 = case shown="True" "Edit temp and Press" {
              frame False {
              }
              frame True {
                n141 = stacked-sequence {
                  frame #0 {
                    w478 = TRUE  # Wait until done
                    n142 = call "Run_Enter_Temp.vi"("Wait until done"=w478) -> ()  [unwired: 1 out]
                  }
                  frame #1 {
                    n143 = call "Get_Temp_and_Press.vi"("Averaging time (mins)"=0.5) -> ("Abs Press (mbar)"=w480:dbl, "Temperature"=w479:dbl)  [unwired: 3 out]
                    n144 = local write "Abs Press (mbar)"(w480) -> ()
                    n145 = local write "Temp (deg C)"(w479) -> ()
                  }
                }
              }
            }
          }
          frame #11 {
            n146 = case shown="False" "OK" {
              tunnel: w484 -> [_ w488]
              tunnel: [TRUE w487] -> w482
              frame False {
              }
              frame True {
                n147 = stacked-sequence {
                  seq-local: [w489 _] -> [_ w507]
                  tunnel: w488 -> [w491 w509]
                  tunnel: [_ w505] -> w487
                  frame #0 {
                    n148 = for {
                      shift-right: [w498] -> _
                      shift-left: i16[] [] -> [w497]
                      tunnel: w491 -> [w494] mode=indexing
                      tunnel: [w493] -> w490 mode=indexing
                      n149 = Unbundle By Name(w494) -> ("Ch No"=w495:i16)
                      n150 = Search 1D Array(1D array=w497, element=w495) -> (index of element=w496:i32)  [unwired: 1 out]
                      n151 = Build Array (concatenate)(w497, w495) -> (w498:i16[])
                      n152 = case shown="0, Default" w496 {
                        tunnel: w495 -> [w503 _]
                        tunnel: [w499 FALSE ("true")] -> w493
                        frame 0, Default {
                          n153 = Format Into String(format string="The Ch No %d appears more than once", w503) -> (resulting string=w501:string)  [unwired: 2 in, 1 out]
                          n154 = One Button Dialog(message=w501, button name ("OK")="Ok") -> (true=w499:bool)
                        }
                        frame -1 {
                        }
                      }
                    }
                    n155 = Or Array Elements(Boolean array=w490) -> (logical OR=w489:bool)
                  }
                  frame #1 {
                    n156 = for {
                      tunnel: w509 -> [w515] mode=indexing
                      tunnel: [w514] -> w508 mode=indexing
                      n157 = Unbundle By Name(w515) -> ("high limit (10V)"=w513:sgl, "low limit (-10V)"=w512:sgl, "Ch No"=w510:i16)
                      n158 = Greater Or Equal?(x=w513, y=w512) -> (x >= y?=w511:bool)
                      n159 = case shown="False" w511 {
                        tunnel: [TRUE ("true") FALSE ("true")] -> w514
                        tunnel: w510 -> [w517 _]
                        frame False {
                          n160 = Number To Decimal String(number=w517) -> (decimal integer string=w518:string)  [unwired: 1 out]
                          n161 = Concatenate Strings("Error in input limits for Channel No ", w518) -> (w519:string)
                          n162 = One Button Dialog(message=w519) -> ()  [unwired: 2 out]
                        }
                        frame True {
                        }
                      }
                    }
                    n163 = Or Array Elements(Boolean array=w508) -> (logical OR=w506:bool)
                    n164 = Or(x=w506, y=w507) -> (x .or. y?=w505:bool)
                  }
                }
              }
            }
          }
          frame #12 {
            n165 = Unbundle By Name(w525) -> ("Ref Instrument type"=w524:T2)
            n166 = Equal?(x=Ref_Inst_type."Preston tube" ("Ref Instrument type"), y=w524) -> (x = y?=w522:bool)
            n167 = property on="Preston tube diammeter in mm" class="DigNum (strict)"("Visible"=w522) -> ()  [unwired: 2 in, 2 out]
          }
        }
      }
      "Instrument type" <- w70
      "Ch & spans" <- w73
      "Calib filename" <- w72
      n168 = global write "Calib_global.vi" "Angle/vel calib file"(w67) -> ()
      n169 = global write "Calib_global.vi" "existing angle calib"(w66) -> ()
    }
    frame #4 {
      n170 = global read "Calib_global.vi" "Pre Setup String"() -> (w530:string)
      n171 = case shown="\"Setup Front Panel\"" w535 {
        tunnel: [w537 w547] -> w534
        tunnel: "Sampling speeds" -> [w537 w549]
        tunnel: [w536 w543] -> w532
        tunnel: "Fixed n" -> [w536 _]
        tunnel: w530 -> [_ w542]
        tunnel: w529 -> [_ _]
        frame "Show Setup", Default {
        }
        frame "Setup Front Panel" {
          n172 = call "Get_value_from_string.vi"("Input string"=w542, "Variable name"="Requested sampling rate") -> ("Status"=w540:enum16{"Char in string", "Char not in string"}, "Value"=w538:dbl)  [unwired: 1 in]
          n173 = case shown="\"Char not in string\"" w540 {
            tunnel: [w551 sgl 100.0 ("Sampling Rate /ch (Hz)")] -> w539
            tunnel: w538 -> [w551 _]
            frame "Char in string" {
            }
            frame "Char not in string" {
            }
          }
          n174 = call "Get_value_from_string.vi"("Input string"=w542, "Variable name"="No of samples") -> ("Value"=w548:dbl)  [unwired: 1 in, 1 out]
          n175 = call "Get_Characters_from_string.vi"("Input string"=w542, "Variable name"="Fixed Coefficient n") -> ("Value"=w545:string)  [unwired: 1 in, 1 out]
          n176 = Bundle By Name(cluster=w549, "Samples /ch"=w548, "Sampling Rate /ch (Hz)"=w539) -> (w547:T5)
          n177 = Equal?(x="TRUE", y=w545) -> (x = y?=w543:bool)
        }
      }
      "Sampling speeds Output" <- w534
      "Fixed n out" <- w532
      n178 = property on="Acquisition Plug in" class="Ring (strict)"() -> ("Strings []"=w527:string[])  [unwired: 2 in, 2 out]
      n179 = Index Array(array=w527, index="Acquisition Plug in") -> (element=w526:string)
      n180 = global write "Meas_global.vi" "Acquisition vi to Run"(w526) -> ()
    }
    frame #5 {
      n181 = property on="Calib filename" class="Path"() -> ("Disabled"=w557:u8)  [unwired: 2 in, 2 out]
      n182 = Equal To 0?(x=w557) -> (x = 0?=w556:bool)
      n183 = local read "Reference instrument"() -> (w555:T7)
      n184 = case shown="True" w556 {
        tunnel: w555 -> [w560 w566]
        tunnel: [w559 w565] -> w554
        tunnel: w553 -> [_ w561]
        frame False {
          n185 = Bundle By Name(cluster=w560, "Calib filename"=path "") -> (w559:T7)
        }
        frame True {
          w562 = FALSE  # Use Latest Calib
          n186 = Unbundle By Name(w566) -> ("Calib filename"=w568:path, "Ref Instrument type"=w564:T2)
          n187 = case shown="\"ADAM Channel\"" w564 {
            tunnel: [Inst_type."Propeller anemometer" ("Inst type") Inst_type."Pressure Transducer" ("Inst type") Inst_type."Pressure Transducer" ("Inst type") Inst_type."Pitot-static tube" ("Inst type") Inst_type."Preston tube" ("Inst type") Inst_type."Generic Linear" ("Inst type") Inst_type."Generic Polynomial" ("Inst type") Inst_type."Thermocouple" ("Inst type") Inst_type."Raw voltage" ("Inst type") Inst_type."Raw voltage" ("Inst type") Inst_type."Raw voltage" ("Inst type")] -> w563
            frame "Propellor anemometer" {
            }
            frame "Pressure Transducer" {
            }
            frame "Raw voltage" {
            }
            frame "Pitot-static tube" {
            }
            frame "Preston tube" {
            }
            frame "Generic Linear" {
            }
            frame "Generic Polynomial" {
            }
            frame "Thermocouple" {
            }
            frame "LDA" {
            }
            frame "Enter Value" {
            }
            frame "ADAM Channel" {
            }
          }
          n188 = case shown="\"Take a New Calibration Point\", Default" w561 {
            tunnel: w568 -> [w569 w573]
            tunnel: [w569 w572] -> w567
            tunnel: w563 -> [_ w571]
            tunnel: w562 -> [_ w570]
            frame "Refit Curve" {
            }
            frame "Take a New Calibration Point", Default {
              n189 = call "Find_calibration_file.vi"("Inst type"=w571, "Use Latest Calib"=w570, "filename"=w573) -> ("filename out"=w572:path)  [unwired: 1 in]
            }
          }
          n190 = Bundle By Name(cluster=w566, "Calib filename"=w567) -> (w565:T7)
        }
      }
      n191 = local write "Reference instrument"(w554) -> ()
    }
    frame #6 {
      n192 = property on="Ref vel for angle calib" class="Clust (strict)"() -> ("Disabled"=w585:u8)  [unwired: 2 in, 2 out]
      n193 = local read "Ref vel for angle calib"() -> (w587:T7)
      n194 = case shown="0" w585 {
        tunnel: w587 -> [w592 w608]
        tunnel: [w591 w607] -> w586
        frame 0 {
          w588 = FALSE  # Use Latest Calib
          n195 = Unbundle By Name(w592) -> ("Calib filename"=w594:path, "Ref Instrument type"=w590:T2)
          n196 = case shown="\"Preston tube\"" w590 {
            tunnel: [Inst_type."Propeller anemometer" ("Inst type") Inst_type."Pressure Transducer" ("Inst type") Inst_type."Pressure Transducer" ("Inst type") Inst_type."Pitot-static tube" ("Inst type") Inst_type."Preston tube" ("Inst type") Inst_type."Generic Linear" ("Inst type") Inst_type."Generic Polynomial" ("Inst type") Inst_type."Thermocouple" ("Inst type") Inst_type."Raw voltage" ("Inst type") Inst_type."Raw voltage" ("Inst type") Inst_type."Raw voltage" ("Inst type")] -> w589
            frame "Propellor anemometer" {
            }
            frame "Pressure Transducer" {
            }
            frame "Raw voltage" {
            }
            frame "Pitot-static tube" {
            }
            frame "Preston tube" {
            }
            frame "Generic Linear" {
            }
            frame "Generic Polynomial" {
            }
            frame "Thermocouple" {
            }
            frame "LDA" {
            }
            frame "Enter Value" {
            }
            frame "ADAM Channel" {
            }
          }
          n197 = call "Find_calibration_file.vi"("Inst type"=w589, "Use Latest Calib"=w588, "filename"=w594) -> ("filename out"=w593:path)  [unwired: 1 in]
          n198 = Bundle By Name(cluster=w592, "Calib filename"=w593) -> (w591:T7)
        }
        frame 1, Default {
          n199 = Bundle By Name(cluster=w608, "Calib filename"=path "") -> (w607:T7)
        }
      }
      n200 = local write "Ref vel for angle calib"(w586) -> ()
    }
    frame #7 {
      w615 = Ref_Inst_type."ADAM Channel" ("Ref Instrument type")
      n201 = local read "Ref vel for angle calib"() -> (w617:T7)
      n202 = global write "Calib_global.vi" "Ref Instrument type"(w612) -> ()
      n203 = property on="Ref vel for angle calib" class="Clust (strict)"() -> ("Disabled"=w610:u8)  [unwired: 2 in, 2 out]
      n204 = Unbundle By Name(w617) -> ("Ref Instrument type"=w616:T2)
      n205 = Equal To 0?(x=w610) -> (x = 0?=w609:bool)
      n206 = Equal?(x=w612, y=w615) -> (x = y?=w614:bool)
      n207 = local read "2nd ref instrument"() -> (w618:T6)
      n208 = Bundle By Name(cluster=w618, "2nd Ref type"=w616, "2nd inst present"=w609) -> (→"2nd ref instrument":T6)
      n209 = case shown="True" w609 {
        tunnel: w616 -> [_ w624]
        tunnel: w615 -> [_ w623]
        tunnel: w614 -> [w619 w621]
        tunnel: [w619 w620] -> w613
        frame False {
        }
        frame True {
          n210 = Equal?(x=w624, y=w623) -> (x = y?=w622:bool)
          n211 = Or(x=w622, y=w621) -> (x .or. y?=w620:bool)
        }
      }
    }
    frame #8 {
      n212 = Equal?(x=Calib_mode."Show Setup" ("Mode"), y=w632) -> (x = y?=w631:bool)
      n213 = And(x=w631, y=w630) -> (x .and. y?=w629:bool)
      n214 = global read "Calib_global.vi" "Pre Setup String"() -> (w628:string)
      n215 = case shown="True" w629 {
        tunnel: [w635 w641] -> w633
        tunnel: w628 -> [w637 w640]
        tunnel: "ADAM Channel name" -> [w636 w639]
        tunnel: [w634 w638] -> w626
        frame False {
          n216 = call "Get_Characters_from_string.vi"("Input string"=w637, "Variable name"=w636) -> ("Value"=w634:string)  [unwired: 1 in, 1 out]
          n217 = call "Characters_to_string.vi"("Characters to write"=w634, "Label for characters"=w636) -> ("Output string"=w635:string)
        }
        frame True {
          n218 = stacked-sequence {
            seq-local: [_ w645 _ _ _ _] -> [_ _ _ w655 _ _]
            seq-local: [_ _ _ w649 _ _] -> [_ _ _ _ _ _]
            seq-local: [_ _ w647 _ _ _] -> [_ _ _ _ _ w665]
            tunnel: [_ _ _ _ _ w664] -> w641
            tunnel: w640 -> [_ _ _ _ _ w660]
            tunnel: w639 -> [_ _ _ _ _ w659]
            tunnel: [_ _ _ _ _ w658] -> w638
            frame #0 {
              n219 = property on="Message" class="Str"("Visible"=TRUE) -> ()  [unwired: 2 in, 2 out]
              "Message" <- "Message\n\nCurrently trying to connect to the server.\n\nPlease Wait"
            }
            frame #1 {
              n220 = Get Date/Time In Seconds() -> (seconds since 1Jan1904=w644:timestamp)
              n221 = To Double Precision Float(number=w644) -> (double precision float=w645:dbl)
            }
            frame #2 {
              n222 = call "Get_ADAM_Ch_names_client.vi"("Channel names set"=Channel_names."Active Only") -> ("Ch names"=w647:string[])
            }
            frame #3 {
              n223 = Get Date/Time In Seconds() -> (seconds since 1Jan1904=w648:timestamp)
              n224 = To Double Precision Float(number=w648) -> (double precision float=w654:dbl)
              n225 = Subtract(x=w654, y=w655) -> (x-y=w653:dbl)
              n226 = Number To Decimal String(number=w653) -> (decimal integer string=w651:string)  [unwired: 1 out]
              n227 = Concatenate Strings("Server took ", w651, " Seconds to respond") -> (w649:string)
            }
            frame #4 {
              n228 = property on="Message" class="Str"("Visible"=FALSE) -> ()  [unwired: 2 in, 2 out]
            }
            frame #5 {
              n229 = call "Get_Characters_from_string.vi"("Input string"=w660, "Variable name"=w659) -> ("Status"=w663:enum16{"Char in string", "Char not in string"}, "Value"=w662:string)  [unwired: 1 in]
              n230 = case shown="\"Char in string\"" w663 {
                tunnel: w662 -> [w666 _]
                tunnel: [w666 "" ("Value")] -> w661
                frame "Char in string" {
                }
                frame "Char not in string" {
                }
              }
              n231 = call "Select_Single_ADAM_Ch.vi"("Desired Ch name (in)"=w661, "Available Ch names"=w665, "Message"="Please Choose Reference Instrument") -> ("Ch Name"=w658:string)  [unwired: 3 out]
              n232 = call "Characters_to_string.vi"("Characters to write"=w658, "Label for characters"=w659) -> ("Output string"=w664:string)
            }
          }
        }
      }
      n233 = global write "Calib_global.vi" "ADAM Channel Name"(w626) -> ()
    }
    frame #9 {
      n234 = local read "2nd ref instrument"() -> (w674:T6)
      n235 = Equal?(x=Calib_mode."Show Setup" ("Mode"), y=w681) -> (x = y?=w680:bool)
      n236 = Unbundle By Name(w674) -> ("2nd Ref type"=w672:T2, "2nd inst present"=w670:bool)
      n237 = global read "Calib_global.vi" "Pre Setup String"() -> (w678:string)
      n238 = Equal?(x=Ref_Inst_type."ADAM Channel" ("2nd Ref type"), y=w672) -> (x = y?=w671:bool)
      n239 = And(x=w671, y=w670) -> (x .and. y?=w669:bool)
      n240 = And(x=w680, y=w669) -> (x .and. y?=w679:bool)
      n241 = case shown="True" w679 {
        tunnel: [w683 w689] -> w668
        tunnel: w678 -> [w685 w688]
        tunnel: "ADAM Channel name for 2nd Ref Instr" -> [w684 w687]
        tunnel: [w682 w686] -> w676
        frame False {
          n242 = call "Get_Characters_from_string.vi"("Input string"=w685, "Variable name"=w684) -> ("Value"=w682:string)  [unwired: 1 in, 1 out]
          n243 = call "Characters_to_string.vi"("Characters to write"=w682, "Label for characters"=w684) -> ("Output string"=w683:string)
        }
        frame True {
          n244 = stacked-sequence {
            seq-local: [_ w693 _ _ _ _] -> [_ _ _ w703 _ _]
            seq-local: [_ _ _ w697 _ _] -> [_ _ _ _ _ _]
            seq-local: [_ _ w695 _ _ _] -> [_ _ _ _ _ w713]
            tunnel: [_ _ _ _ _ w712] -> w689
            tunnel: w688 -> [_ _ _ _ _ w708]
            tunnel: w687 -> [_ _ _ _ _ w707]
            tunnel: [_ _ _ _ _ w706] -> w686
            frame #0 {
              n245 = local write "Message"("Message\n\nCurrently trying to connect to the server.\n\nPlease Wait") -> ()
              n246 = property on="Message" class="Str"("Visible"=TRUE) -> ()  [unwired: 2 in, 2 out]
            }
            frame #1 {
              n247 = Get Date/Time In Seconds() -> (seconds since 1Jan1904=w692:timestamp)
              n248 = To Double Precision Float(number=w692) -> (double precision float=w693:dbl)
            }
            frame #2 {
              n249 = call "Get_ADAM_Ch_names_client.vi"("Channel names set"=Channel_names."Active Only") -> ("Ch names"=w695:string[])
            }
            frame #3 {
              n250 = Get Date/Time In Seconds() -> (seconds since 1Jan1904=w696:timestamp)
              n251 = To Double Precision Float(number=w696) -> (double precision float=w702:dbl)
              n252 = Subtract(x=w702, y=w703) -> (x-y=w701:dbl)
              n253 = Number To Decimal String(number=w701) -> (decimal integer string=w699:string)  [unwired: 1 out]
              n254 = Concatenate Strings("Server took ", w699, " Seconds to respond") -> (w697:string)
            }
            frame #4 {
              n255 = property on="Message" class="Str"("Visible"=FALSE) -> ()  [unwired: 2 in, 2 out]
            }
            frame #5 {
              n256 = call "Get_Characters_from_string.vi"("Input string"=w708, "Variable name"=w707) -> ("Status"=w711:enum16{"Char in string", "Char not in string"}, "Value"=w710:string)  [unwired: 1 in]
              n257 = case shown="\"Char in string\"" w711 {
                tunnel: w710 -> [w714 _]
                tunnel: [w714 "" ("Value")] -> w709
                frame "Char in string" {
                }
                frame "Char not in string" {
                }
              }
              n258 = call "Select_Single_ADAM_Ch.vi"("Desired Ch name (in)"=w709, "Available Ch names"=w713, "Message"="Please Choose 2nd Ref Channel") -> ("Ch Name"=w706:string)  [unwired: 3 out]
              n259 = call "Characters_to_string.vi"("Characters to write"=w706, "Label for characters"=w707) -> ("Output string"=w712:string)
            }
          }
        }
      }
      n260 = global write "Calib_global.vi" "ADAM Channel Name Vel Ref"(w676) -> ()
    }
    frame #10 {
      n261 = local read "Reference instrument"() -> (w720:T7)
      n262 = local read "2nd ref instrument"() -> (w721:T6)
      n263 = local read "Sampling speeds Output"() -> (w717:T5)
      n264 = local read "Abs Press (mbar)"() -> (w718:dbl)
      n265 = local read "Temp (deg C)"() -> (w716:dbl)
      n266 = global write "Calib_global.vi" "2nd ref instrument"(w721) -> ()
      n267 = Unbundle By Name(w717) -> ("Sampling Rate /ch (Hz)"=w723:sgl, "Samples /ch"=w724:i32)
      n268 = global write "Calib_global.vi" "Abs Press (mbar)"(w718) -> ()
      n269 = global write "Calib_global.vi" "Temp (deg C)"(w716) -> ()
      n270 = call "Calib_General_Setup.vi"("Reference instrument"=w720, "Requested No of samples"=w724, "Sampling rate (Hz)"=w723, "2nd ref instrument"=w721, "Temp"=w716, "Abs Press (mbar)"=w718) -> ("Output string"=w722:string, "LDA Data"=w719:bool)  [unwired: 8 out]
    }
    frame #11 {
      n271 = local read "Ref vel for angle calib"() -> (w733:T7)
      n272 = local read "Reference instrument"() -> (w732:T7)
      n273 = local read "Instrument type"() -> (w731:T8)
      n274 = global write "Calib_global.vi" "Instrument type"(w731) -> ()
      n275 = case shown="\"Propeller anemometer\", Default" w731 {
        tunnel: [w736 w737 w739] -> w730
        tunnel: w733 -> [w735 w738 _]
        tunnel: [w735 w738 w739] -> w726
        tunnel: w732 -> [w736 w737 w739]
        frame "Propeller anemometer", Default {
        }
        frame "Cross wire angle" {
        }
        frame "Cross wire velocity" {
        }
      }
      n276 = call "Reference_Inst_Info_2_string.vi"("Reference instrument"=w730, "Reference Name"="Reference instrument") -> ("Setup String"=w728:string)
      n277 = call "Reference_Inst_Info_2_string.vi"("Reference instrument"=w726, "Reference Name"="Ref vel for angle calib") -> ("Setup String"=w725:string)
      n278 = Concatenate Strings(w728, w725) -> (w734:string)
    }
    frame #12 {
      n279 = local read "Instrument type"() -> (w740:T8)
      n280 = case shown="\"Pulsed Wire\"" w740 {
        tunnel: ["" w749] -> w741
        tunnel: w742 -> [_ w748]
        frame "Propeller anemometer", Default {
        }
        frame "Pulsed Wire" {
          w744 = FALSE  # Check Calib file?
          n281 = case shown="\"Refit Curve\", Default" w748 {
            tunnel: [w751 w753] -> w747
            tunnel: [w750 w752] -> w746
            frame "Refit Curve", Default {
              w751 = FALSE  # Show Panel?
              w750 = T13 TRUE  # OK
            }
            frame "Show Setup" {
              w753 = TRUE  # Show Panel?
              w752 = T13 FALSE  # OK
            }
          }
          n282 = global read "Calib_global.vi" "Pre Setup String"() -> (w745:string)
          n283 = call "PWA_Setup_Panel.vi"("Show Panel?"=w747, "Check Calib file?"=w744, "OK"=w746, "Incoming Setup String"=w745) -> ("Outgoing Setup String"=w749:string)  [unwired: 3 out]
        }
      }
    }
    frame #13 {
      n284 = local read "instrument to calibrate"() -> (w756:T10)
      n285 = for {
        tunnel: w756 -> [w783] mode=indexing
        shift-right: [w768] -> w759
        shift-left: "" -> [w772]
        i -> [w782]
        n286 = Unbundle By Name(w783) -> ("high limit (10V)"=w779:sgl, "low limit (-10V)"=w774:sgl, "Ch No"=w773:i16)
        n287 = Increment(x=w782) -> (x+1=w767:i32)
        n288 = Format Into String(format string="Inst_to_calibrate_element_%d ", w767) -> (resulting string=w765:string)  [unwired: 2 in, 1 out]
        n289 = Concatenate Strings(w765, "Low limit") -> (w778:string)
        n290 = Concatenate Strings(w765, "Ch No") -> (w777:string)
        n291 = Concatenate Strings(w765, "High limit") -> (w780:string)
        n292 = call "Value_to_string.vi"("Value"=w774, "Label for value"=w778) -> ("Output string"=w770:string)  [unwired: 1 in]
        n293 = call "Value_to_string.vi"("Value"=w773, "Label for value"=w777) -> ("Output string"=w769:string)  [unwired: 1 in]
        n294 = call "Value_to_string.vi"("Value"=w779, "Label for value"=w780) -> ("Output string"=w771:string)  [unwired: 1 in]
        n295 = Concatenate Strings(w772, w771, w770, w769) -> (w768:string)
      }
      n296 = Array Size(array=w756) -> (size(s)=w755:i32)
      n297 = Equal To 0?(x=w755) -> (x = 0?=w754:bool)
      n298 = case shown="True" w754 {
        tunnel: [w761 i16 -10 ("Ch No")] -> w757
        tunnel: w756 -> [w760 _]
        frame False {
          w763 = 0  # index
          n299 = Index Array(array=w760, index=w763) -> (element=w762:T19)
          n300 = Unbundle By Name(w762) -> ("Ch No"=w761:i16)
        }
        frame True {
        }
      }
      n301 = global write "Calib_global.vi" "Calib Ch No"(w757) -> ()
    }
    frame #14 {
      n302 = local read "Preston tube diammeter in mm"() -> (w787:dbl)
      n303 = local read "Instrument type"() -> (w798:T8)
      n304 = property on="Instrument type" class="Enum (strict)"() -> ("Strings []"=w799:string[])  [unwired: 2 in, 2 out]
      n305 = local read "angle calib"() -> (w792:T9)
      n306 = property on="angle calib" class="Enum (strict)"() -> ("Strings []"=w793:string[])  [unwired: 2 in, 2 out]
      n307 = Index Array(array=w799, index=w798) -> (element=w797:string)
      n308 = Index Array(array=w793, index=w792) -> (element=w791:string)
      n309 = call "Characters_to_string.vi"("Characters to write"=w797, "Label for characters"="Instrument_type_to Calibrate") -> ("Output string"=w795:string)
      n310 = call "Value_to_string.vi"("Value"=w787, "Label for value"="Preston tube diameter in mm" ("Variable name")) -> ("Output string"=w786:string)  [unwired: 1 in]
      n311 = call "Characters_to_string.vi"("Characters to write"=w791, "Label for characters"="Angle calib") -> ("Output string"=w790:string)
      n312 = local read "Fixed n out"() -> (w803:bool)
      n313 = Concatenate Strings(w786, w795, w790) -> (w810:string)
      n314 = Select(t="TRUE", s=w803, f="FALSE") -> (s? t:f=w804:string)
      n315 = global read "Calib_global.vi" "New Setup String"() -> (w802:string)
      n316 = call "Characters_to_string.vi"("Characters to write"=w804, "Label for characters"="Fixed Coefficient n") -> ("Output string"=w800:string)
      n317 = Concatenate Strings(w802, w800, w810, w809, w784, w808, w785, w801, w789) -> (w811:string)
      n318 = global write "Calib_global.vi" "New Setup String"(w811) -> ()
    }
    frame #15 {
      n319 = Equal?(x=Calib_mode."Show Setup" ("Mode"), y=w817) -> (x = y?=w816:bool)
      n320 = And(x=w815, y=w816) -> (x .and. y?=w814:bool)
      n321 = case shown="True" w814 {
        tunnel: [FALSE ("Synchronise with LDA") FALSE ("Synchronise with LDA")] -> w812
        frame False {
        }
        frame True {
          n322 = global read "LDA_meas_global_1.vi" "BSA Type"() -> (w821:T20)
          n323 = case shown="\"57N11\"" w821 {
            tunnel: TRUE -> [_ w831]
            frame "57N11" {
              n324 = stacked-sequence {
                frame #0 {
                  n325 = Bundle By Name(cluster=T17 {"dimensions"=enum."2D", "Analogue Freq Multiplier"=0.1} ("LDA set up"), "dimensions"=enum16{"1D", "2D"}."1D", "Analogue Freq Multiplier"=2.0) -> (w824:T17)
                  n326 = global write "Meas_global.vi" "LDA set up"(w824) -> ()
                }
                frame #1 {
                  w826 = "1"  # BSA Number
                  n327 = call "Control_BSA_setup.vi"("setup"=Setup."Show Setup", "BSA number"=w826) -> ()  [unwired: 14 out]
                }
                frame #2 {
                  n328 = global read "LDA_meas_global_2.vi" "BSA2 info"() -> (w828:T21)
                  n329 = Unbundle By Name(w828) -> ("GPIB Address"=w829:string)
                  n330 = call "Set_BSA_Coincidence.vi"("GPIB address"=w829, "Set Coincidence"=enum16{"Slave", "Master", "Private"}."Slave") -> ()  [unwired: 1 in, 5 out]
                }
              }
            }
            frame "BSA F60" {
              n331 = disable-structure shown="TARGET_TYPE==Windows" {
                disable-tunnel: w831 -> [_ w832]
                frame condition #0 {
                }
                frame condition #1 (active) {
                  n332 = call "Edit_BSA_IP.vi"("Show Panel"=w832) -> ()  [unwired: 3 out]
                }
              }
            }
          }
        }
      }
      n333 = global write "Meas_global.vi" "Synchronise with LDA"(w812) -> ()
    }
    frame #16 {
      w840 = TRUE  # Lock File
      w850 = FALSE  # advisory dialog? (display:T)
      w851 = FALSE  # append to file? (new file:F)
      n334 = local read "Calib filename"() -> (w852:path)
      n335 = local read "Instrument type"() -> (w838:T8)
      n336 = global read "Meas_global.vi" "LDA data"() -> (w843:enum16{"No LDA data", "Take LDA data"})
      n337 = global write "Calib_global.vi" "Ref Calib file"(w852) -> ()
      n338 = local read "Ch & spans"() -> (w844:T12)
      n339 = case shown="\"Take LDA data\"" w843 {
        tunnel: ["" w861] -> w841
        frame "No LDA data" {
        }
        frame "Take LDA data" {
          w860 = ""  # Used to be LDA-header.vi
          n340 = call "LDA_U16_data_header.vi"() -> ("Output string"=w862:string)  [unwired: 1 out]
          n341 = Concatenate Strings(w860, w862) -> (w861:string)
        }
      }
      n342 = case shown="\"Pulsed Wire\"" w838 {
        tunnel: ["" w854] -> w837
        frame "Propeller anemometer", Default {
        }
        frame "Pulsed Wire" {
          n343 = property on="PWA Data" class="Enum (strict)"() -> ("Strings []"=w857:string[])  [unwired: 2 in, 2 out]
          n344 = Index Array(array=w857, index=PWA_Data."One Ch PWA" ("PWA Data")) -> (element=w855:string)
          n345 = call "Characters_to_string.vi"("Characters to write"=w855, "Label for characters"="Pulsed_Wire_Data" ("Variable name")) -> ("Output string"=w854:string)
        }
      }
      n346 = call "Calib_Ch_setup.vi"("Preston tube diammeter in mm"="Preston tube diammeter in mm", "Ch & spans"=w844, "Calib filename"=w852) -> ("Output string"=w845:string)
      n347 = global write "Calib_global.vi" "Ch & spans"(w844) -> ()
      n348 = call "Date_and_Time_to_string.vi"() -> ("Date and time (spreadsheet)"=w842:string)
      n349 = Concatenate Strings(w842, w837, w841, w846, w845, w836) -> (w847:string)
      n350 = call "Setup_Filepath.vi"("Setup File Type"=Setup_Filetype."Measurement Setups", "Filename in"="Calib_Setup.xls") -> ("Filename Out"=w833:path)  [unwired: 1 out]
      n351 = call "Add_label_to_string.vi"("String to write"=w847, "File Label"="Raw data header") -> ("Output string"=w848:string)
      n352 = call "Write_Characters_To_File.vi"("file path (dialog if empty)"=w833, "advisory dialog? (display:T)"=w850, "character string"=w848, "append to file? (new file:F)"=w851, "Lock File"=w840) -> ()  [unwired: 4 out]
    }
    frame #17 {
      n353 = case shown="\"Show Setup\"" w863 {
        frame "Show Setup" {
          n354 = Current VI's Path() -> (path=w865:path)
          n355 = call "Open_Close_Front_Panel.ph.vi"("Front Panel Window:Open"=FALSE, "VI path"=w865) -> ()  [unwired: 2 out]
        }
        frame "Take a New Calibration Point", Default {
        }
      }
    }
  }
